vi "HTML_Tags_Create_IMG_Element.vi"(9 "Table css-Attributes[]":string[][](array[string]), 10 "Image Path/Name":string) -> (2 "IMG Element":string)   [LabVIEW 2014]
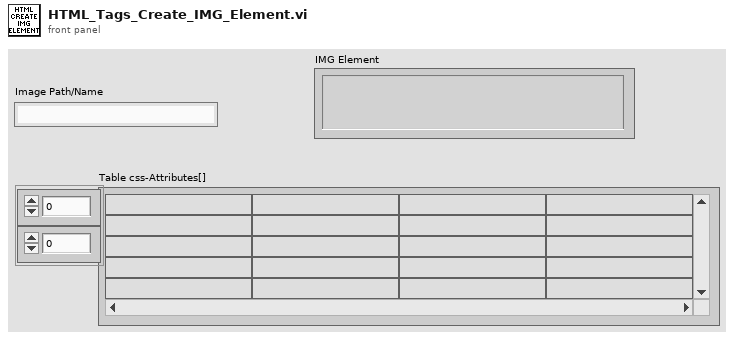
[diagram p1: front panel]
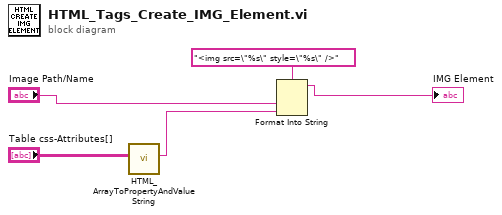
[diagram p0: block diagram]
diagram:
  n1 = call "HTML_ArrayToPropertyAndValueString.vi"("Table css-Attributes[]"="Table css-Attributes[]") -> ("spreadsheet string"=w2:string)  [unwired: 10 in]
  n2 = Format Into String(format string="<img src=\"%s\" style=\"%s\" />", "Image Path/Name", w2) -> (resulting string=→"IMG Element":string)  [unwired: 2 in, 1 out]
